vi "Read-Write Text File.vi"(5 "Team Files Folder":path, 6 "Read(f) Save(t)":bool, 7 "File Name":string, 8 "Error":errorcluster, 11 "Text Data":string) -> (0 "Error Out":errorcluster, 2 "Success Out":bool, 3 "Text Data Out":string)   [LabVIEW 2020]
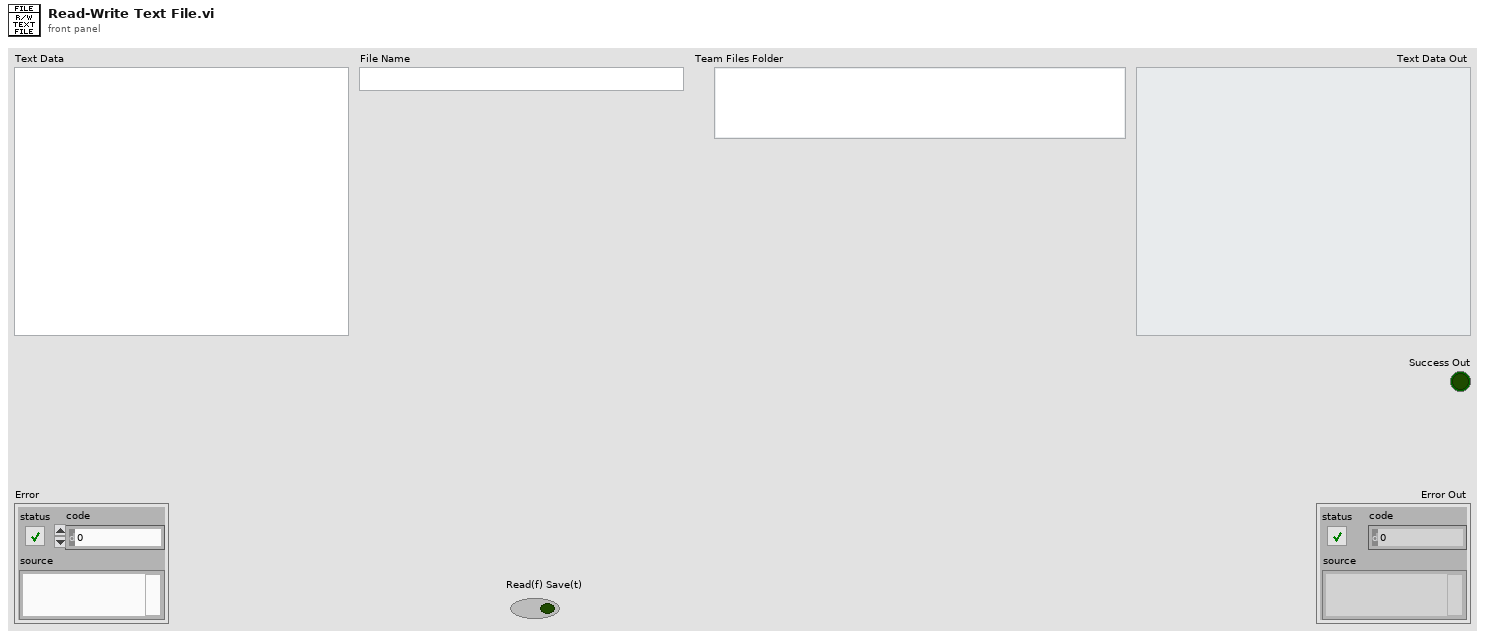
[diagram p1: front panel]
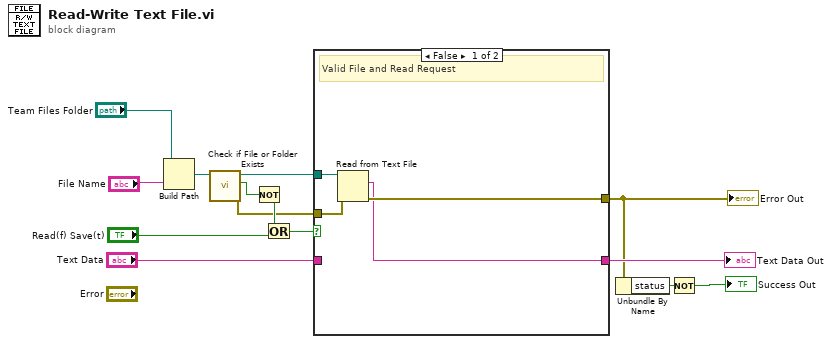
[diagram p0: block diagram]
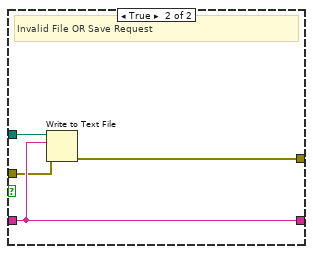
[diagram p2: hidden frame]
diagram:
  n1 = Build Path(base path="Team Files Folder", name or relative path="File Name") -> (appended path=w8:path)
  n2 = call <vilib>:"Check if File or Folder Exists.vi"("path"=w8) -> ("error out"=w2:errorcluster, "file or folder exists?"=w4:bool, "dup path"=w7:path)  [unwired: 8 in]
  n3 = Not(x=w4) -> (.not. x?=w3:bool)
  n4 = Or(x=w3, y="Read(f) Save(t)") -> (x .or. y?=w5:bool)
  n5 = case shown="False" w5 {
    tunnel: w7 -> [w16 w22]
    tunnel: "Text Data" -> [_ w20]
    tunnel: [w18 w21] -> w10
    tunnel: [w17 w20] -> w11
    tunnel: w2 -> [w15 w19]
    frame False {
      # "Valid File and Read Request"
      n6 = Read from Text File(file (use dialog)=w16, error in=w15) -> (text=w17:string, error out=w18:errorcluster)  [unwired: 2 in, 2 out]
    }
    frame True {
      # "Invalid File OR Save Request"
      n7 = Write to Text File(file (use dialog)=w22, text=w20, error in=w19) -> (error out=w21:errorcluster)  [unwired: 1 in, 2 out]
    }
  }
  "Text Data Out" <- w11
  "Error Out" <- w10
  n8 = Unbundle By Name(w10) -> ("status"=w9:bool)
  n9 = Not(x=w9) -> (.not. x?=→"Success Out":bool)
